vi "Get NI MAX Info.vi"(8 "error in (no error)":errorcluster) -> (0 "error out":errorcluster, 3 "Device Info":T1[](array[typedef]))   [LabVIEW 2020, in "Instrument Detection.lvlib"]
doc: "Extracts NI MAX info regarding the connected instruments."
uses:
  Instrument Detection.lvlib
  Controls/Ctl_NI MAX Device Info.ctl
  PPL/HDH.Actor Framework.Core.Instrument Driver.lvlibp/Instrument Driver/Controls/Ctl_ConnectionType.ctl
  <vilib>/nisyscfg/Close (Filter).vi
  <vilib>/nisyscfg/Close (System).vi
  <vilib>/nisyscfg/Close (Resources).vi
  <vilib>/nisyscfg/nisyscfg.lvlib
  <resource>/objmgr/nisysapi.rc
  PPL/HDH.Actor Framework.Core.Instrument Driver.lvlibp/Instrument Driver/Instrument Driver.lvclass
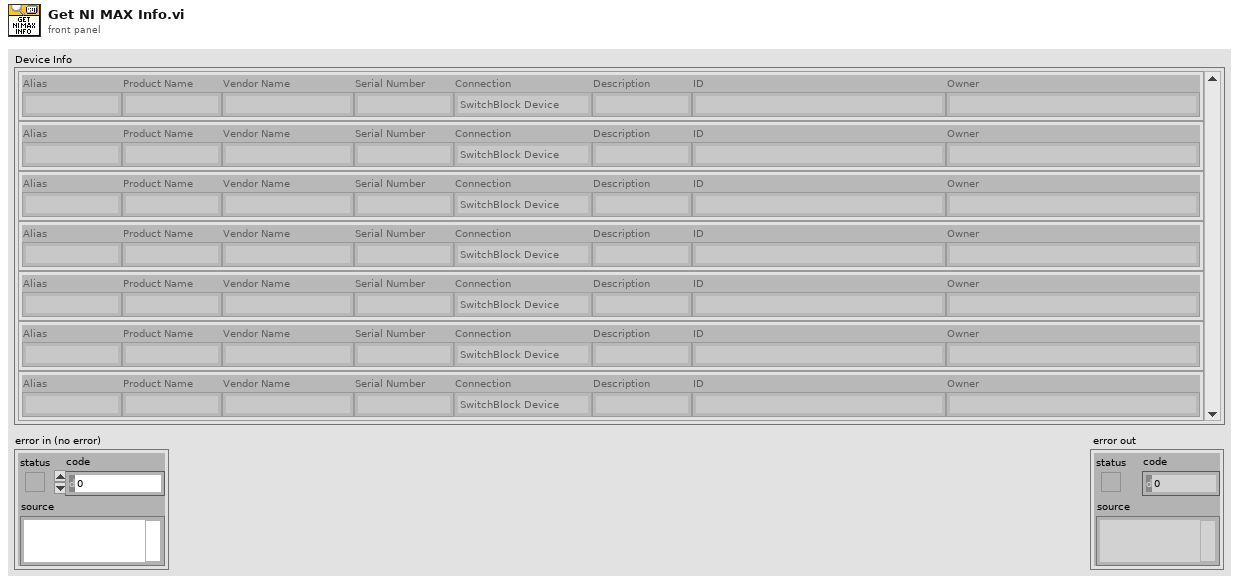
[diagram p1: front panel]
types:
  T1 = typedef "Instrument Detection.lvlib/Ctl_NI MAX Device Info.ctl" = cluster{"Alias":string, "Product Name":string, "Vendor Name":string, "Serial Number":string, "Connection":T2, "Description":string, "ID":string, "Owner":string}
  T2 = typedef "HDH.Actor Framework.Core.Instrument Driver.lvlibp/Instrument Driver.lvclass/Ctl_ConnectionType.ctl" = enum16{"BuiltIn/System", "PXI/PCI", "USB", "GPIB", "VXI", "Serial", "TCP/IP", "cRIO", "SCXI", "cDAQ", "SwitchBlock", "SCC", "FireWire", "Accessory", "CAN", "SwitchBlock Device"}
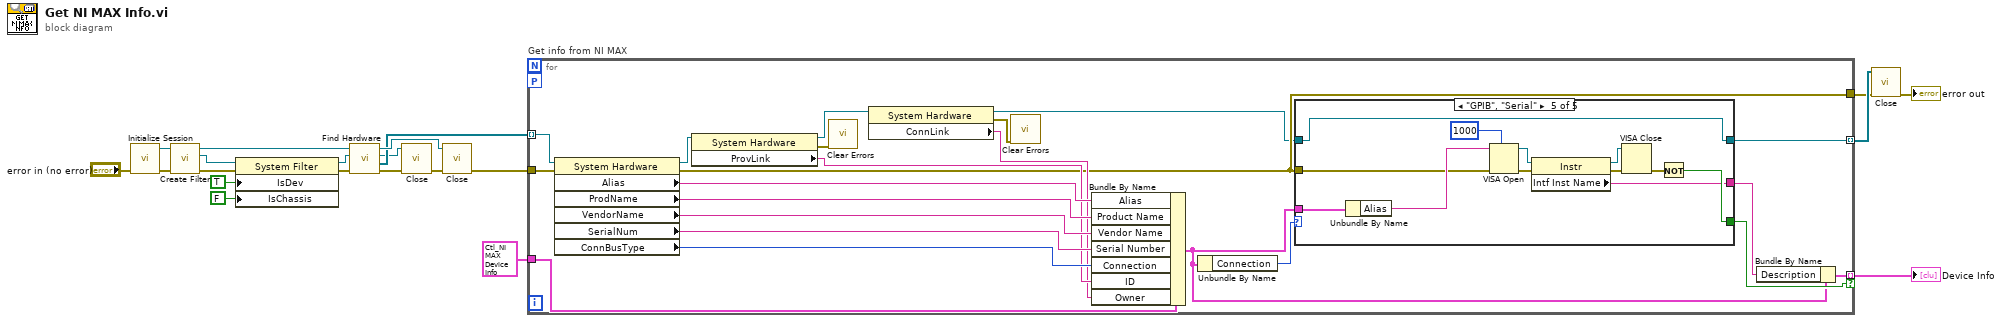
[diagram p0: block diagram]
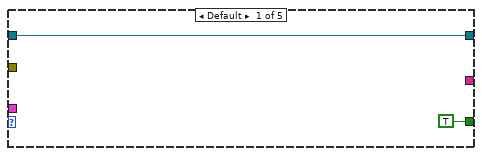
[diagram p2: hidden frame]
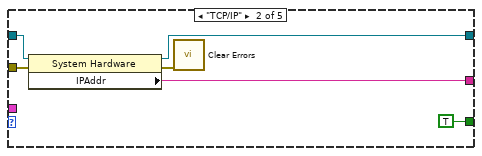
[diagram p3: hidden frame]
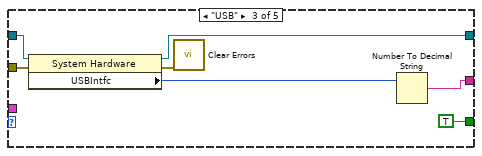
[diagram p4: hidden frame]
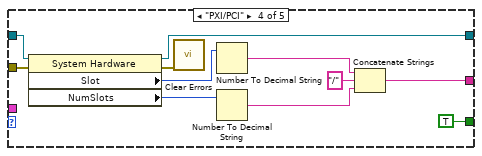
[diagram p5: hidden frame]
diagram:
  n1 = call <vilib>:"Initialize Session.vi"("error in (no error)"="error in (no error)") -> ("error out"=w8:errorcluster, "Session out"=w12:refnum<k21>)  [unwired: 9 in]
  n2 = call <vilib>:"Create Filter.vi"("error in (no error)"=w8, "Session in"=w12) -> ("error out"=w16:errorcluster, "Filter out"=w15:refnum<k20>, "Session out"=w1:refnum<k21>)  [unwired: 7 in]
  n3 = property class="System Filter"(reference=w15, error in=w16, "IsDev"=TRUE ("Is Device"), "IsChassis"=FALSE ("Is Chassis")) -> (reference out=w13:refnum<k20>, error out=w7:errorcluster)
  n4 = call <vilib>:"Find Hardware.vi"("error in (no error)"=w7, "Filter in"=w13, "Session in"=w1) -> ("error out"=w10:errorcluster, "Resources out"=w20:refnum<k20>[], "Filter out"=w11:refnum<k20>, "Session out"=w21:refnum<k21>)  [unwired: 5 in]
  n5 = call-poly <vilib>:"Close.vi"("error in (no error)"=w10, "Filter in"=w11) -> ("error out"=w9:errorcluster)  [unwired: 9 in]
  n6 = call-poly <vilib>:"Close.vi"("error in (no error)"=w9, "Session in"=w21) -> ("error out"=w18:errorcluster)  [unwired: 9 in]
  n7 = for "Get info from NI MAX" {
    tunnel: w20 -> [w43] mode=indexing
    tunnel: [w25] -> w19 mode=indexing
    tunnel: T1 {"Alias"="", "Product Name"="", "Vendor Name"="", "Serial Number"="", "Connection"=enum."SwitchBlock Device", "Description"="", "ID"="", "Owner"=""} ("Instrument Detection.lvlib:Ctl_NI MAX Device Info") -> [w41]
    workers-P: _ -> [_]
    tunnel: w18 -> [w42]
    tunnel: [w27] -> w17
    tunnel: [w23] -> w3 mode=indexing if=w28
    n8 = property class="System Hardware"(reference=w43, error in=w42) -> (reference out=w30:refnum<k20>, error out=w27:errorcluster, "Alias"=w40:string, "ProdName"=w39:string, "VendorName"=w38:string, "SerialNum"=w37:string, "ConnBusType"=w36:u32)
    n9 = property class="System Hardware"(reference=w30) -> (reference out=w35:refnum<k20>, error out=w32:errorcluster, "ProvLink"=w34:string)  [unwired: 1 in]
    n10 = call <vilib>:"Clear Errors.vi"("error in (no error)"=w32) -> ()  [unwired: 5 in, 2 out]
    n11 = property class="System Hardware"(reference=w35) -> (reference out=w26:refnum<k20>, error out=w31:errorcluster, "ConnLink"=w33:string)  [unwired: 1 in]
    n12 = call <vilib>:"Clear Errors.vi"("error in (no error)"=w31) -> ()  [unwired: 5 in, 2 out]
    n13 = Bundle By Name(cluster=w41, "Alias"=w40, "Product Name"=w39, "Vendor Name"=w38, "Serial Number"=w37, "Connection"=w36, "ID"=w34, "Owner"=w33) -> (w24:T1)
    n14 = Unbundle By Name(w24) -> ("Connection"=w29:T2)
    n15 = case shown="\"GPIB\", \"Serial\"" w29 {
      tunnel: [_ w50 w52 w61 w70] -> w22
      tunnel: w24 -> [_ _ _ _ w76]
      tunnel: [TRUE TRUE TRUE TRUE w77] -> w28
      tunnel: w27 -> [_ w49 w56 w67 w75]
      tunnel: [w44 w47 w54 w65 w71] -> w25
      tunnel: w26 -> [w44 w51 w58 w69 w71]
      frame Default {
      }
      frame "TCP/IP" {
        n16 = property class="System Hardware"(reference=w51, error in=w49) -> (reference out=w47:refnum<k20>, error out=w48:errorcluster, "IPAddr"=w50:string)
        n17 = call <vilib>:"Clear Errors.vi"("error in (no error)"=w48) -> ()  [unwired: 5 in, 2 out]
      }
      frame "USB" {
        n18 = property class="System Hardware"(reference=w58, error in=w56) -> (reference out=w54:refnum<k20>, error out=w55:errorcluster, "USBIntfc"=w57:u32)
        n19 = call <vilib>:"Clear Errors.vi"("error in (no error)"=w55) -> ()  [unwired: 5 in, 2 out]
        n20 = Number To Decimal String(number=w57) -> (decimal integer string=w52:string)  [unwired: 1 in]
      }
      frame "PXI/PCI" {
        n21 = property class="System Hardware"(reference=w69, error in=w67) -> (reference out=w65:refnum<k20>, error out=w66:errorcluster, "Slot"=w68:i32, "NumSlots"=w62:i32)
        n22 = call <vilib>:"Clear Errors.vi"("error in (no error)"=w66) -> ()  [unwired: 5 in, 2 out]
        n23 = Number To Decimal String(number=w68) -> (decimal integer string=w63:string)  [unwired: 1 in]
        n24 = Number To Decimal String(number=w62) -> (decimal integer string=w60:string)  [unwired: 1 in]
        n25 = Concatenate Strings(w63, "/" ("string"), w60) -> (w61:string)
      }
      frame "GPIB", "Serial" {
        n26 = Unbundle By Name(w76) -> ("Alias"=w81:string)
        n27 = VISA Open(timeout (0)=u32 1000 ("VISA Open timeout (0)"), error in (no error)=w75, VISA resource name=w81) -> (VISA resource name=w80:refnum<visa-resource-name>, error out=w74:errorcluster)  [unwired: 2 in]
        n28 = property class="Instr"(reference=w80, error in=w74) -> (reference out=w79:refnum<visa-resource-name>, error out=w73:errorcluster, "Intf Inst Name"=w70:string)
        n29 = VISA Close(VISA resource name=w79, error in (no error)=w73) -> (error out=w78:errorcluster)
        n30 = Not(x=w78) -> (.not. x?=w77:bool)
      }
    }
    n31 = Bundle By Name(cluster=w24, "Description"=w22) -> (w23:T1)
  }
  "Device Info" <- w3
  n32 = call-poly <vilib>:"Close.vi"("error in (no error)"=w17, "Resources in"=w19) -> ("error out"=→"error out":errorcluster)  [unwired: 9 in]
